vi "Close DVR Referance.vi"(8 "error in (no error)":errorcluster, 11 "Addr. Mode DVR":refnum<data-value>) -> (0 "error out":errorcluster)   [LabVIEW 2020, in "Addressing Mode.lvclass"]
uses:
  Addressing Mode.lvclass
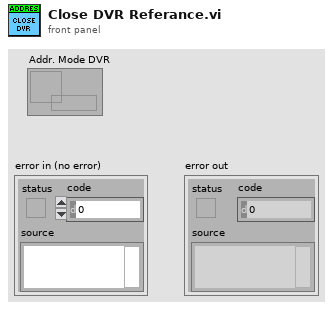
[diagram p1: front panel]
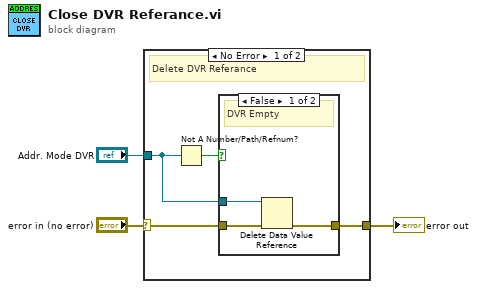
[diagram p0: block diagram]
diagram:
  n1 = case shown="No Error" "error in (no error)" {
    selector: "error in (no error)" -> [w6 w12]
    tunnel: [w7 w12] -> w2
    tunnel: "Addr. Mode DVR" -> [w4 _]
    frame No Error {
      # "Delete DVR Referance"
      n2 = Not A Number/Path/Refnum?(number/path/refnum=w4) -> (NaN/Path/Refnum?=w5:bool)
      n3 = case shown="False" w5 {
        tunnel: [w9 w11] -> w7
        tunnel: w6 -> [w10 w11]
        tunnel: w4 -> [w8 _]
        frame False {
          # "DVR Empty"
          n4 = Delete Data Value Reference(data value reference=w8, error in=w10) -> (error out=w9:errorcluster)  [unwired: 1 out]
        }
        frame True {
        }
      }
    }
    frame Error {
    }
  }
  "error out" <- w2
